vi "addLink.vi"(4 "arguments":string[](array[string]), 6 "executablePath":string, 8 "Error In":errorcluster, 9 "title":string, 10 "icon":refnum<class "QIcon.lvclass">, 11 "QWinJumpListCategory In":refnum<class "QWinJumpListCategory.lvclass">) -> (0 "Error Out":errorcluster, 2 "Value":refnum<class "QWinJumpListItem.lvclass">, 3 "QWinJumpListCategory Out":refnum<class "QWinJumpListCategory.lvclass">)   [LabVIEW 2014, in "QWinJumpListCategory.lvclass"]
doc: "LabVIEW-specific documentation is not yet available. See <b>https://doc.qt.io/qt-5/qwinjumplistcategory.html#addLink</b>"
uses:
  QWinJumpListCategory.lvclass
  QWinJumpListItem/QWinJumpListItem.lvclass
  Qt GUI/QIcon/QIcon.lvclass
  LQ Core/LQIdentity/LQIdentity.lvclass/LQIdentity.ctl
  LQ Core/LQSerialData/LQSerialData.lvclass/LQSerialData.ctl
  LQ Core/LQ Core.lvlib
  LQ Core/LQIdentity/LQIdentity.lvclass
  LQ Core/LQCoreEngine/LQCoreEngine.lvclass
  LQ Core/LQSerialData/LQSerialData.lvclass
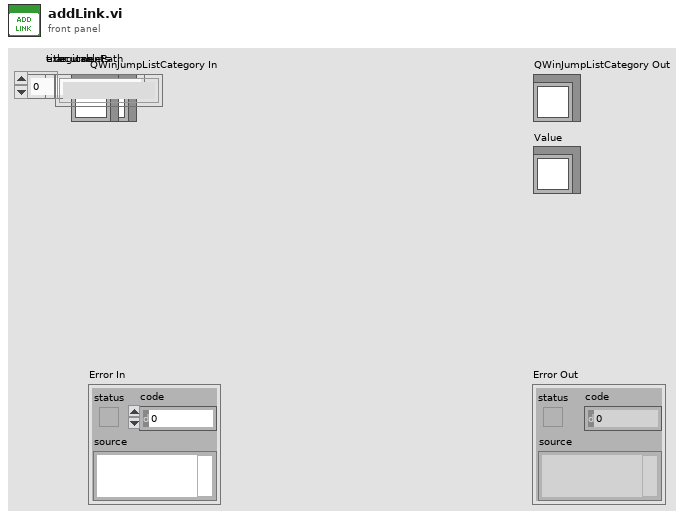
[diagram p1: front panel]
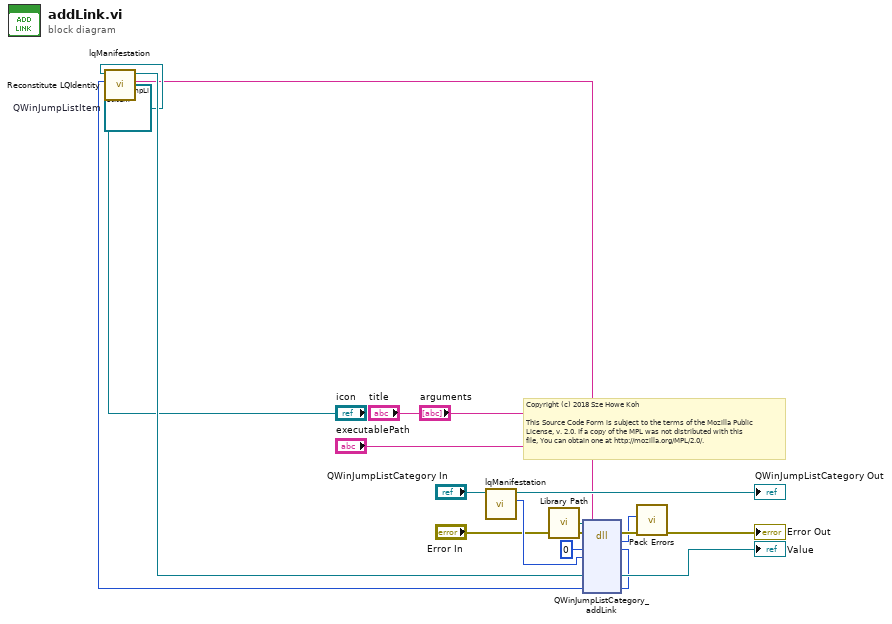
[diagram p0: block diagram]
diagram:
  w6 = refnum<class "QWinJumpListItem.lvclass"> refnum  # QWinJumpListItem
  # "Copyright (c) 2018 Sze Howe Koh\n\nThis Source Code Form is subject to the terms of the Mozilla Public\nLicense, v. 2.0. If a copy of the MPL was not distributed with this\nfile, You can obtain one at http://mozilla.org/MPL/2.0/."
  n1 = call "lqManifestation.vi"("LQSerialData in"="icon") -> ("Manifestation"=w4:string)  [unwired: 9 in, 1 out]
  n2 = call "lqManifestation.vi"("LQIdentity in"="QWinJumpListCategory In") -> ("Manifestation"=w13:u64, "LQIdentity out"=→"QWinJumpListCategory Out":refnum<class "QWinJumpListCategory.lvclass">)  [unwired: 9 in]
  n3 = call "Library Path.vi"() -> ("Library Path"=w14:path)
  n4 = dll-call lib="?" fn="QWinJumpListCategory_addLink"(path in=w14, error in="Error In", "_retVal"=u64 0 ("retVal"), "_instance"=w13, "icon"=w4, "title"="title", "executablePath"="executablePath", "arguments"="arguments") -> (error out=w11:errorcluster, w9:i32, "_retVal"=w7:u64)  [unwired: 6 in, 1 out]
  n5 = call "Reconstitute LQIdentity.vi"("Manifestation"=w7, "LQIdentity Prototype"=w6) -> ("Reconstituted LQIdentity"=→"Value":refnum<class "QWinJumpListItem.lvclass">)  [unwired: 8 in, 1 out]
  n6 = call "Pack Errors.vi"("Error In"=w11, "Error Code"=w9) -> ("Error Out"=→"Error Out":errorcluster)  [unwired: 9 in]
